vi "Crop Video Time.vi"() -> ()   [LabVIEW 2017]
uses:
  <vilib>/vision/NI_Vision_Development_Module.lvlib
  <vilib>/userdefined/High Color/IMAQdx.ctl
  <vilib>/vision/Image Controls.llb/IMAQ Image.ctl
  <vilib>/vision/Avi.llb/IMAQ AVI2 Refnum.ctl
  WEISS-Ultrasound-Frame-Grabber/LabVIEW/Controls/Position.ctl
  WEISS-Ultrasound-Frame-Grabber/LabVIEW/Controls/Orientation.ctl
  WEISS-Ultrasound-Frame-Grabber/LabVIEW/Controls/Rigid Body Info.ctl
  WEISS-Ultrasound-Frame-Grabber/LabVIEW/Controls/Refnums.ctl
  WEISS-Ultrasound-Frame-Grabber/LabVIEW/Controls/Room Dimensions.ctl
  WEISS-Ultrasound-Frame-Grabber/LabVIEW/Controls/Dimensions.ctl
  WEISS-Ultrasound-Frame-Grabber/LabVIEW/Controls/Frame Grabber Data.ctl
  WEISS-Ultrasound-Frame-Grabber/LabVIEW/Controls/Recording Settings.ctl
  WEISS-Ultrasound-Frame-Grabber/LabVIEW/Controls/Operator.ctl
  WEISS-Ultrasound-Frame-Grabber/LabVIEW/Controls/Operator Settings.ctl
panel:
  in  "Crop Outside":bool
  in  "Play":bool
  in  "Frame Slider":cluster{u32, u32, u32}(slide)={162, 79, 57} scale=0.0..179.0
  in  "Codec":u16(ring)=3 items=["Cinepak Codec by Radius", "Intel IYUV codec", "Microsoft Video 1", "FF Video Codec 1 (FFV1) (NI Vision)", "Motion JPEG (NI Vision)", "Y800 Uncompressed Grey Scale (NI Vision)", "YUV 4:2:0 Planar (NI Vision)"]
  out "Saving":bool
  in  "Display?":bool
  in  "Crop Inside":bool
  in  "Stop":bool
  out "Video path":path
  out "Crop ROI":i32[](array[numeric])
  in  "Frame Grabber Data":T1={"Camera Session"="", "Frame"=refnum, "AVI Refnum"=refnum, "Codecs"=[], "Frame number"=0, "Tracking File Refnum"=refnum, "Tick Count"=0, "Probe Object"=refnum, "Playback Probe Data"=[], "Rigid Body"={"Position"={"x (mm)"=0.0, "y (mm)"=0.0, "z (mm)"=0.0}, "Orientation"={"Pitch (rad)"=0.0, "Yaw (rad)"=0.0, "Roll (rad)"=0.0}, "Quaternion"={"qx"=0.0, "qy"=0.0, "qz"=0.0, "qw"=0.0}, "Tracked?"=FALSE}, "Total no frames playback"=0, "Video FPS"=0.0, "Camera connected?"=FALSE, "Scene"=refnum, "Cropped Frame"=refnum, "Tracker FPS"=0.0, "Crop ROI"=[], "Presentation Values"=[], "Elapsed time (ms)"=0, "Camera frames playback"=0, "Refnums"={"Live Refnum"=refnum, "Record Refnum"=refnum, "Recording Settings Refnum"=refnum, "Playback Refnum"=refnum, "Frame Slider Refnum"=refnum, "Pause Refnum"=refnum, "Home Refnum"=refnum, "Crop Refnum"=refnum, "Clear Crop Refnum"=refnum, "stop refnum"=refnum, "Playback Rate Refnum"=refnum, "Operator Settings Refnums"=refnum, "Presentation Refnum"=refnum, "Gestation Refnum"=refnum, "Connection Settings Refnum"=refnum}, "Dimensions"={"Probe Dimensions"={"Probe Width"=0.0, "Probe Depth"=1.0, "Probe Height"=0.0}, "Room Dimensions"={"Room Width"=0.0, "Room Depth"=0.0, "Room Height"=0.0}}}
  in  "Save":bool
  in  "Open":bool
  out "Frame":T3(plugin-control)
  # "Frame"
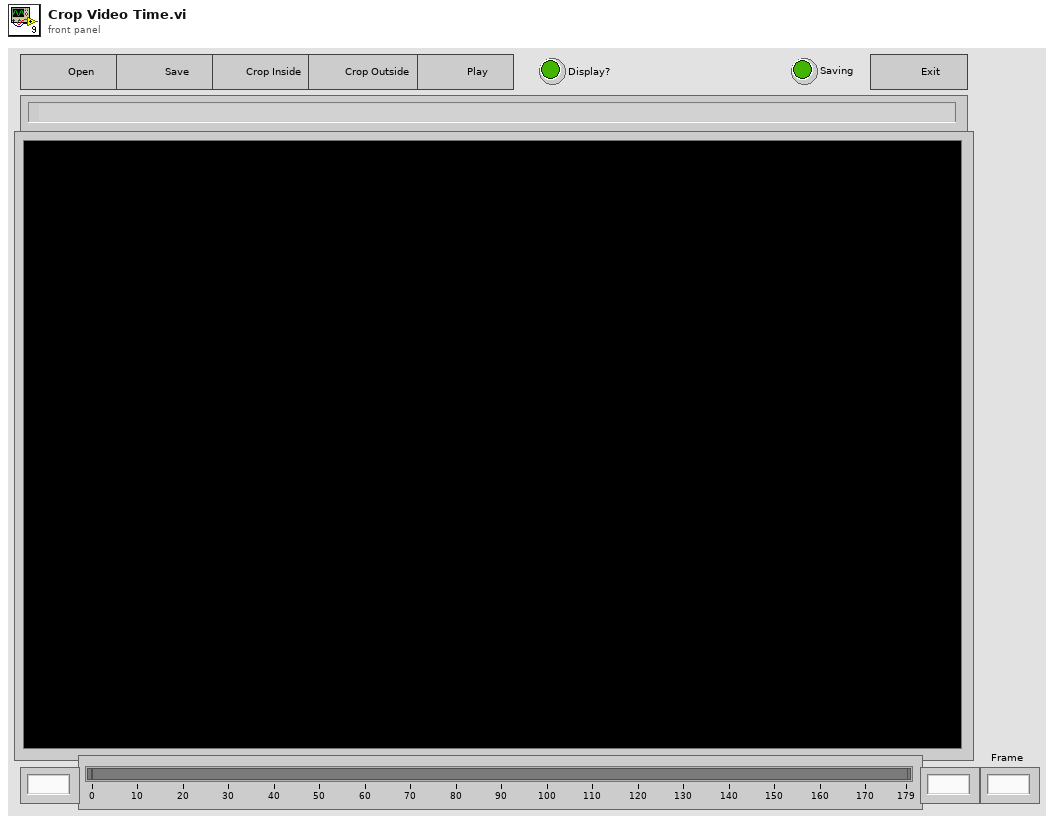
[diagram p1: front panel]
types:
  T1 = typedef "Frame Grabber Data.ctl" = cluster{"Camera Session":T2, "Frame":T3, "AVI Refnum":T4, "Codecs":string[], "Frame number":u32, "Tracking File Refnum":refnum<file>, "Tick Count":u32, "Probe Object":refnum<vi>, "Playback Probe Data":dbl[][], "Rigid Body":T5, "Total no frames playback":i32, "Video FPS":dbl, "Camera connected?":bool, "Scene":refnum<vi>, "Cropped Frame":T3, "Tracker FPS":dbl, "Crop ROI":i32[], "Presentation Values":string[], "Elapsed time (ms)":u32, "Camera frames playback":u32, "Refnums":T8, "Dimensions":T9}
  T2 = typedef "IMAQdx.ctl" = refnum<k21>
  T3 = typedef "IMAQ Image.ctl" = refnum<image>
  T4 = typedef "IMAQ AVI2 Refnum.ctl" = refnum<k20>
  T5 = typedef "Rigid Body Info.ctl" = cluster{"Position":T6, "Orientation":T7, "Quaternion":cluster{"qx":sgl, "qy":sgl, "qz":sgl, "qw":sgl}, "Tracked?":bool}
  T6 = typedef "Position.ctl" = cluster{"x (mm)":sgl, "y (mm)":sgl, "z (mm)":sgl}
  T7 = typedef "Orientation.ctl" = cluster{"Pitch (rad)":sgl, "Yaw (rad)":sgl, "Roll (rad)":sgl}
  T8 = typedef "Refnums.ctl" = cluster{"Live Refnum":refnum<vi>, "Record Refnum":refnum<vi>, "Recording Settings Refnum":refnum<vi>, "Playback Refnum":refnum<vi>, "Frame Slider Refnum":refnum<vi>, "Pause Refnum":refnum<vi>, "Home Refnum":refnum<vi>, "Crop Refnum":refnum<vi>, "Clear Crop Refnum":refnum<vi>, "stop refnum":refnum<vi>, "Playback Rate Refnum":refnum<vi>, "Operator Settings Refnums":refnum<vi>, "Presentation Refnum":refnum<vi>, "Gestation Refnum":refnum<vi>, "Connection Settings Refnum":refnum<vi>}
  T9 = typedef "Dimensions.ctl" = cluster{"Probe Dimensions":cluster{"Probe Width":sgl, "Probe Depth":sgl, "Probe Height":sgl}, "Room Dimensions":T10}
  T10 = typedef "Room Dimensions.ctl" = cluster{"Room Width":dbl, "Room Depth":dbl, "Room Height":dbl}
  T11 = enum16{"Init", "Wait", "Load", "Playback", "Crop Inside", "Crop Outside", "Shutdown"}
  T12 = enum8{"Enabled", "Disabled", "Disabled and Grayed Out"}
  T13 = typedef "Image Type" = u32
  T14 = enum16{"open", "replace", "create", "open or create", "replace or create", "replace or create with confirmation"}
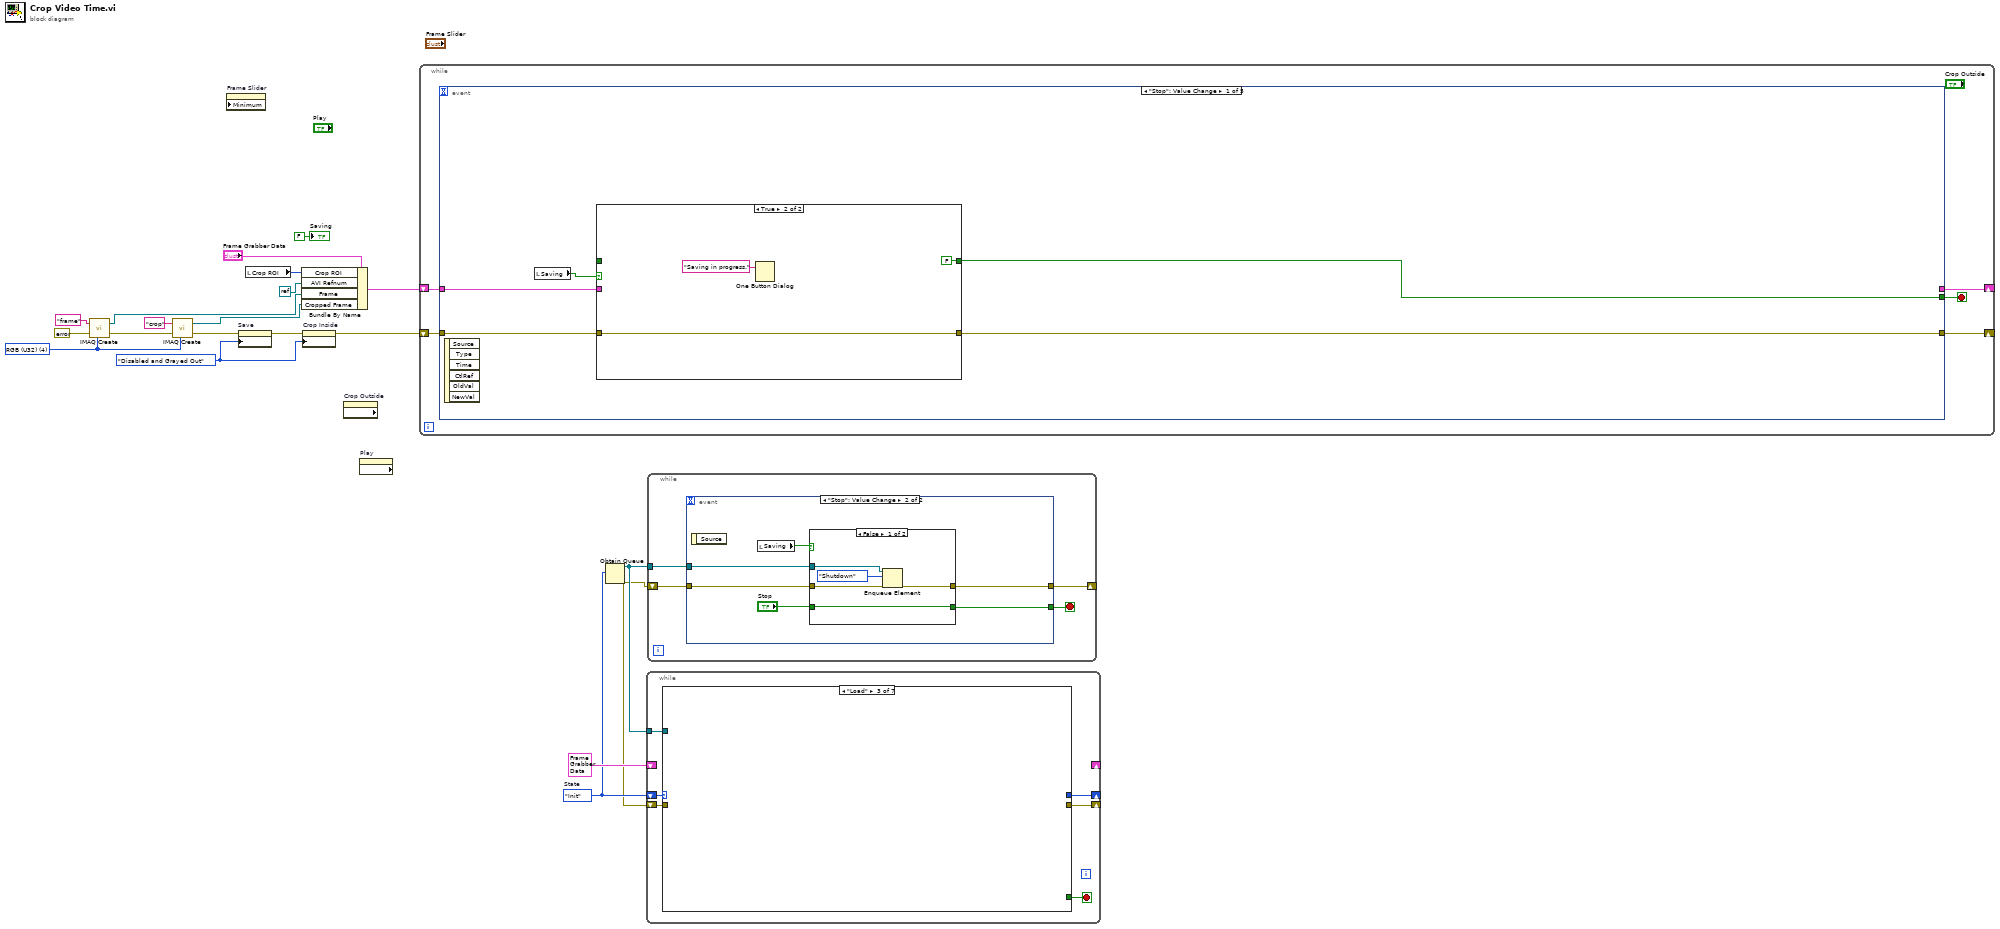
[diagram p0: block diagram]
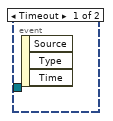
[diagram p2: hidden frame]
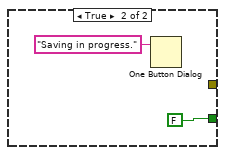
[diagram p3: hidden frame]
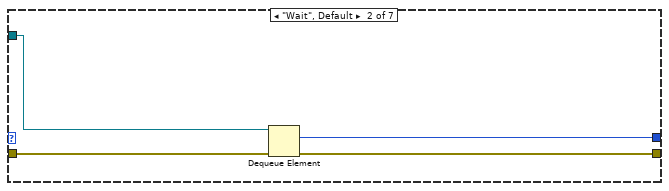
[diagram p5: hidden frame]
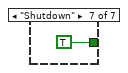
[diagram p9: hidden frame]
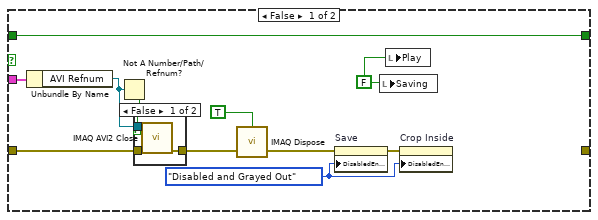
[diagram p10: hidden frame]
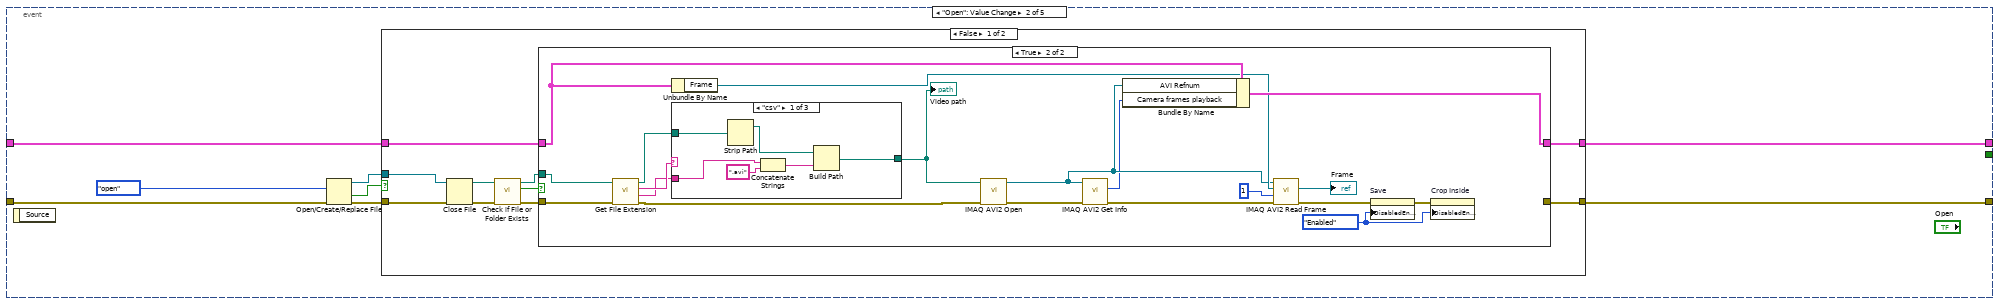
[diagram p12: hidden frame]
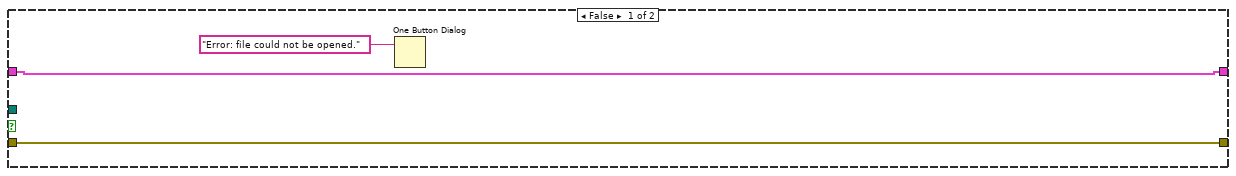
[diagram p13: hidden frame]
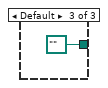
[diagram p15: hidden frame]
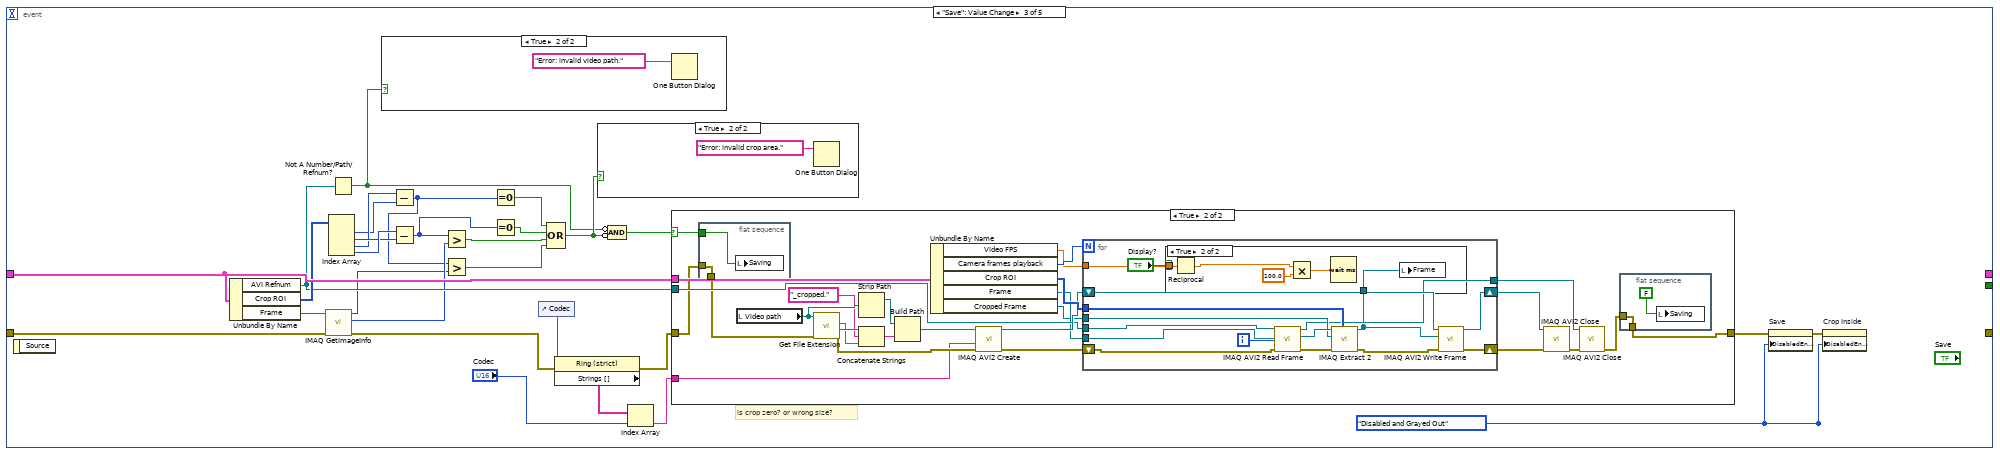
[diagram p17: hidden frame]
diagram:
  w3 = T11."Init"  # State
  w7 = T12."Disabled and Grayed Out" ("Disabled")
  w12 = T13 4 items=["Grayscale (U8)", "Grayscale (I16)", "Grayscale (SGL)", "Complex (CSG)", "RGB (U32)", "HSL (U32)", "RGB (U64)", "Grayscale (U16)"] ("Image Type")
  n1 = call "IMAQ Create"("Image Name"="frame", "Image Type"=w12, "error in (no error)"=errorcluster {"status"=FALSE, "code"=0, "source"=""}) -> ("New Image"=w15:T3, "error out"=w13:errorcluster)  [unwired: 2 in]
  n2 = call "IMAQ Create"("Image Name"="crop", "Image Type"=w12, "error in (no error)"=w13) -> ("New Image"=w16:T3, "error out"=w9:errorcluster)  [unwired: 2 in]
  n3 = property on="Frame Slider" class="Slide (strict)" props=["Minimum"]() -> ()  [unwired: 3 in, 2 out]
  n4 = property on="Save" class="Bool"(error in=w9, "DisabledEnum"=w7) -> (error out=w8:errorcluster)  [unwired: 1 in, 1 out]
  n5 = local read "Crop ROI"() -> (w10:i32[])
  n6 = Bundle By Name(cluster="Frame Grabber Data", "Crop ROI"=w10, "AVI Refnum"=refnum<k0> refnum, "Frame"=w15, "Cropped Frame"=w16) -> (w19:T1)
  n7 = property on="Crop Inside" class="Bool"(error in=w8, "DisabledEnum"=w7) -> (error out=w5:errorcluster)  [unwired: 1 in, 1 out]
  n8 = property on="Crop Outside" class="Bool" props=["DisabledEnum"]() -> ()  [unwired: 2 in, 3 out]
  n9 = property on="Play" class="Bool (strict)" props=["DisabledEnum"]() -> ()  [unwired: 2 in, 3 out]
  n10 = while {
    shift-right: [w22] -> _
    shift-left: w19 -> [w23]
    shift-right: [w21] -> _
    shift-left: w5 -> [w24]
    stop <- w25 stop-if-true
    n11 = event shown="[0] \"Stop\": Value Change" {
      selector: _ -> [_ _ _ _ _]
      dyn-events: _ -> [_ _ _ _ _]
      timeout: _ -> [_ _ _ _ _]
      tunnel: [w26 _ _ _ _] -> w25
      tunnel: w24 -> [w30 w57 w116 w189 w193]
      tunnel: w23 -> [w29 w52 w129 w190 w196]
      tunnel: [_ w51 _ w188 w191] -> w22
      tunnel: [w28 w50 w108 w185 w192] -> w21
      event "Stop": Value Change {
        n12 = event-data() -> ()  [unwired: 1 in, 6 out]
        n13 = local read "Saving"() -> (w27:bool)
        n14 = case shown="True" w27 {
          tunnel: w30 -> [w42 w48]
          tunnel: w29 -> [w41 _]
          tunnel: [w37 w48] -> w28
          tunnel: _ -> [w32 _]
          tunnel: [w32 FALSE ("Stop")] -> w26
          frame False {
            w31 = FALSE
            w35 = T12."Disabled and Grayed Out" ("Disabled")
            n15 = Unbundle By Name(w41) -> ("AVI Refnum"=w34:T4)
            n16 = Not A Number/Path/Refnum?(number/path/refnum=w34) -> (NaN/Path/Refnum?=w33:bool)
            n17 = case shown="False" w33 {
              tunnel: w42 -> [w45 w46]
              tunnel: [w44 w46] -> w39
              tunnel: w34 -> [w43 _]
              frame False {
                n18 = call "IMAQ AVI2 Close"("error in (no error)"=w45, "AVI Refnum"=w43) -> ("error out"=w44:errorcluster)  [unwired: 9 in]
              }
              frame True {
              }
            }
            n19 = call "IMAQ Dispose"("All Images? (No)"=TRUE, "error in (no error)"=w39) -> ("error out"=w38:errorcluster)  [unwired: 4 in]
            n20 = property on="Save" class="Bool"(error in=w38, "DisabledEnum"=w35) -> (error out=w36:errorcluster)  [unwired: 1 in, 1 out]
            n21 = local write "Saving"(w31) -> ()
            n22 = local write "Play"(w31) -> ()
            n23 = property on="Crop Inside" class="Bool"(error in=w36, "DisabledEnum"=w35) -> ()  [unwired: 1 in, 2 out]
          }
          frame True {
            n24 = One Button Dialog(message="Saving in progress.") -> ()  [unwired: 1 in, 1 out]
          }
        }
      }
      event "Open": Value Change {
        n25 = event-data() -> ()  [unwired: 1 in, 1 out]
        n26 = Open/Create/Replace File(error in=w57, operation (0:open)=T14."open") -> (refnum out=w53:refnum<file>, cancelled=w56:bool, error out=w54:errorcluster)  [unwired: 4 in]
        n27 = case shown="False" w56 {
          tunnel: w54 -> [w64 w98]
          tunnel: w53 -> [w65 _]
          tunnel: w52 -> [w61 w99]
          tunnel: [w60 w99] -> w51
          tunnel: [w58 w98] -> w50
          frame False {
            n28 = Close File(refnum=w65, error in=w64) -> (path=w62:path, error out=w63:errorcluster)
            n29 = call <vilib>:"Check if File or Folder Exists.vi"("error in (no error)"=w63, "path"=w62) -> ("error out"=w67:errorcluster, "file or folder exists?"=w59:bool, "dup path"=w66:path)  [unwired: 7 in]
            n30 = case shown="True" w59 {
              tunnel: w67 -> [w69 w77]
              tunnel: w66 -> [_ w73]
              tunnel: w61 -> [w70 w88]
              tunnel: [w70 w89] -> w60
              tunnel: [w69 _] -> w58
              frame False {
                n31 = One Button Dialog(message="Error: file could not be opened.") -> ()  [unwired: 1 in, 1 out]
              }
              frame True {
                w78 = T12."Enabled" ("Disabled")
                n32 = call <vilib>:"Get File Extension.vi"("error in (no error)"=w77, "file"=w73) -> ("error out"=w76:errorcluster, "filename without extension"=w74:string, "lowercase file extension"=w75:string, "dup file"=w72:path)  [unwired: 5 in, 1 out]
                n33 = Unbundle By Name(w88) -> ("Frame"=w87:T3)
                n34 = case shown="\"csv\"" w75 {
                  tunnel: w74 -> [w95 _ _]
                  tunnel: [w90 w96 path "" ("dup file")] -> w71
                  tunnel: w72 -> [w91 w96 _]
                  frame "csv" {
                    n35 = Strip Path(path=w91) -> (stripped path=w93:path)  [unwired: 1 out]
                    n36 = Concatenate Strings(w95, ".avi" ("string")) -> (w92:string)
                    n37 = Build Path(base path=w93, name or relative path=w92) -> (appended path=w90:path)
                  }
                  frame "avi" {
                  }
                  frame Default {
                  }
                }
                "Video path" <- w71
                n38 = call "IMAQ AVI2 Open"("error in (no error)"=w76, "AVI File Path"=w71) -> ("error out"=w83:errorcluster, "AVI Refnum"=w84:T4)  [unwired: 8 in]
                n39 = call "IMAQ AVI2 Get Info"("error in (no error)"=w83, "AVI Refnum"=w84) -> ("error out"=w82:errorcluster, "Number of Frames"=w81:u32)  [unwired: 5 in, 3 out]
                n40 = Bundle By Name(cluster=w88, "AVI Refnum"=w84, "Camera frames playback"=w81) -> (w89:T1)
                n41 = call "IMAQ AVI2 Read Frame"("error in (no error)"=w82, "Frame Number"=u32 1, "Image"=w87, "AVI Refnum"=w84) -> ("error out"=w80:errorcluster, "Image Out"=→"Frame":T3)  [unwired: 5 in, 1 out]
                n42 = property on="Save" class="Bool"(error in=w80, "DisabledEnum"=w78) -> (error out=w79:errorcluster)  [unwired: 1 in, 1 out]
                n43 = property on="Crop Inside" class="Bool"(error in=w79, "DisabledEnum"=w78) -> ()  [unwired: 1 in, 2 out]
              }
            }
          }
          frame True {
          }
        }
      }
      event "Save": Value Change {
        w106 = T12."Disabled and Grayed Out" ("Disabled")
        # "is crop zero? or wrong size?"
        n44 = event-data() -> ()  [unwired: 1 in, 1 out]
        n45 = Unbundle By Name(w129) -> ("AVI Refnum"=w117:T4, "Crop ROI"=w122:i32[], "Frame"=w115:T3)
        n46 = call "IMAQ GetImageInfo"("error in (no error)"=w116, "Image"=w115) -> ("error out"=w105:errorcluster, "Y Resolution"=w114:i32, "X Resolution"=w112:i32)  [unwired: 2 in, 5 out]
        n47 = Index Array(array=w122) -> (element #1=w123:i32, element #2=w125:i32, element #3=w124:i32, element #4=w126:i32)  [unwired: 4 in]
        n48 = Not A Number/Path/Refnum?(number/path/refnum=w117) -> (NaN/Path/Refnum?=w118:bool)
        n49 = case shown="True" w118 {
          frame False {
          }
          frame True {
            n50 = One Button Dialog(message="Error: invalid video path.") -> ()  [unwired: 1 in, 1 out]
          }
        }
        n51 = Subtract(x=w124, y=w123) -> (x-y=w111:i32)
        n52 = Subtract(x=w126, y=w125) -> (x-y=w109:i32)
        n53 = Greater?(x=w109, y=w114) -> (0:w113:bool)
        n54 = Greater?(x=w111, y=w112) -> (0:w110:bool)
        n55 = Equal To 0?(x=w111) -> (x = 0?=w127:bool)
        n56 = Equal To 0?(x=w109) -> (x = 0?=w128:bool)
        n57 = control-ref of="Codec"() -> (w103:refnum<vi>)
        n58 = Compound Arithmetic op=OR(w127, w128, w113, w110) -> (w119:bool)
        n59 = property class="Ring (strict)"(reference=w103, error in=w105) -> (error out=w104:errorcluster, "Strings []"=w101:string[])  [unwired: 1 out]
        n60 = case shown="True" w119 {
          frame False {
          }
          frame True {
            n61 = One Button Dialog(message="Error: invalid crop area.") -> ()  [unwired: 1 in, 1 out]
          }
        }
        n62 = Compound Arithmetic op=AND(invert w118, invert w119) -> (w120:bool)
        n63 = Index Array(array=w101, index="Codec") -> (element=w100:string)
        n64 = case shown="True" w120 {
          selector: w120 -> [_ w138]
          tunnel: w129 -> [_ w159]
          tunnel: w117 -> [_ w146]
          tunnel: [w132 w134] -> w121
          tunnel: w104 -> [w132 w137]
          tunnel: w100 -> [_ w133]
          frame False {
          }
          frame True {
            n65 = flat-sequence {
              tunnel: w138 -> [w163]
              tunnel: w137 -> [w162]
              tunnel: [w162] -> w136
              frame #0 {
                n66 = local write "Saving"(w163) -> ()
              }
            }
            n67 = local read "Video path"() -> (w154:path)
            n68 = call <vilib>:"Get File Extension.vi"("error in (no error)"=w136, "file"=w154) -> ("error out"=w155:errorcluster, "filename without extension"=w152:string, "lowercase file extension"=w150:string)  [unwired: 5 in, 2 out]
            n69 = Strip Path(path=w154) -> (stripped path=w153:path)  [unwired: 1 out]
            n70 = Concatenate Strings(w152, "_cropped." ("string"), w150) -> (w149:string)
            n71 = Build Path(base path=w153, name or relative path=w149) -> (appended path=w148:path)
            n72 = Unbundle By Name(w159) -> ("Video FPS"=w139:dbl, "Camera frames playback"=w158:u32, "Crop ROI"=w157:i32[], "Frame"=w145:T3, "Cropped Frame"=w144:T3)
            n73 = call "IMAQ AVI2 Create"("error in (no error)"=w155, "Codec"=w133, "AVI Path"=w148) -> ("error out"=w147:errorcluster, "AVI Refnum"=w156:T4)  [unwired: 7 in]
            n74 = for {
              N: w158 -> [_]
              shift-right: [w174] -> w143
              shift-left: w147 -> [w178]
              tunnel: w157 -> [w177]
              tunnel: w146 -> [w173]
              tunnel: w145 -> [w172]
              tunnel: w144 -> [w170]
              shift-right: [w169] -> w142
              shift-left: w156 -> [w176]
              tunnel: [w168] -> w140
              tunnel: w139 -> [w165]
              i -> [w179]
              n75 = call "IMAQ AVI2 Read Frame"("error in (no error)"=w178, "Frame Number"=w179, "Image"=w172, "AVI Refnum"=w173) -> ("error out"=w166:errorcluster, "Image Out"=w171:T3, "AVI Refnum (duplicate)"=w168:T4)  [unwired: 5 in]
              n76 = call "IMAQ Extract 2"("Optional Rectangle"=w177, "error in (no error)"=w166, "Image Dst"=w170, "Image Src"=w171) -> ("error out"=w175:errorcluster, "Image Dst Out"=w167:T3)  [unwired: 6 in]
              n77 = case shown="True" "Display?" {
                tunnel: w167 -> [_ w184]
                tunnel: w165 -> [_ w183]
                frame False {
                }
                frame True {
                  n78 = Reciprocal(x=w183) -> (1/x=w182:dbl)
                  n79 = Multiply(x=w182, y=100.0) -> (x*y=w180:dbl)
                  n80 = Wait (ms)(milliseconds to wait=w180) -> ()  [unwired: 1 out]
                  n81 = local write "Frame"(w184) -> ()
                }
              }
              n82 = call "IMAQ AVI2 Write Frame"("error in (no error)"=w175, "Image"=w167, "AVI Refnum"=w176) -> ("error out"=w174:errorcluster, "AVI Refnum (duplicate)"=w169:T4)  [unwired: 6 in, 1 out]
            }
            n83 = call "IMAQ AVI2 Close"("error in (no error)"=w143, "AVI Refnum"=w142) -> ("error out"=w141:errorcluster)  [unwired: 9 in]
            n84 = call "IMAQ AVI2 Close"("error in (no error)"=w141, "AVI Refnum"=w140) -> ("error out"=w135:errorcluster)  [unwired: 9 in]
            n85 = flat-sequence {
              tunnel: w135 -> [w161]
              tunnel: [w161] -> w134
              frame #0 {
                n86 = local write "Saving"(FALSE) -> ()
              }
            }
          }
        }
        n87 = property on="Save" class="Bool"(error in=w121, "DisabledEnum"=w106) -> (error out=w107:errorcluster)  [unwired: 1 in, 1 out]
        n88 = property on="Crop Inside" class="Bool"(error in=w107, "DisabledEnum"=w106) -> ()  [unwired: 1 in, 2 out]
      }
      event "Crop Inside": Value Change {
        n89 = event-data() -> ()  [unwired: 1 in, 1 out]
        n90 = call "Set Crop ROI.vi"("error in (no error)"=w189, "Frame Grabber Data in"=w190) -> ("error out"=w185:errorcluster, "Crop ROI"=→"Crop ROI":i32[], "Image Out"=w187:T3, "Frame Grabber Data out"=w188:T1)  [unwired: 6 in]
        n91 = local write "Frame"(w187) -> ()
      }
      event #4 (no event record) {
        n92 = event-data() -> ()  [unwired: 1 in, 1 out]
        n93 = call "Clear Crop ROI.vi"("error in (no error)"=w193, "Frame Grabber Data in"=w196) -> ("error out"=w192:errorcluster, "Image Out"=w195:T3, "Crop ROI"=w194:i32[], "Frame Grabber Data out"=w191:T1)  [unwired: 6 in]
        n94 = local write "Frame"(w195) -> ()
        n95 = local write "Crop ROI"(w194) -> ()
      }
    }
  }
  n96 = Obtain Queue(element data type=w3) -> (queue out=w2:refnum<queue>, error out=w1:errorcluster)  [unwired: 4 in, 1 out]
  n97 = while {
    shift-right: _ -> [_]
    shift-left: T1 {"Camera Session"="", "Frame"=refnum, "AVI Refnum"=refnum, "Codecs"=[], "Frame number"=0, "Tracking File Refnum"=refnum, "Tick Count"=0, "Probe Object"=refnum, "Playback Probe Data"=[], "Rigid Body"={"Position"={"x (mm)"=0.0, "y (mm)"=0.0, "z (mm)"=0.0}, "Orientation"={"Pitch (rad)"=0.0, "Yaw (rad)"=0.0, "Roll (rad)"=0.0}, "Quaternion"={"qx"=0.0, "qy"=0.0, "qz"=0.0, "qw"=0.0}, "Tracked?"=FALSE}, "Total no frames playback"=0, "Video FPS"=0.0, "Camera connected?"=FALSE, "Scene"=refnum, "Cropped Frame"=refnum, "Tracker FPS"=0.0, "Crop ROI"=[], "Presentation Values"=[], "Elapsed time (ms)"=0, "Camera frames playback"=0, "Refnums"={"Live Refnum"=refnum, "Record Refnum"=refnum, "Recording Settings Refnum"=refnum, "Playback Refnum"=refnum, "Frame Slider Refnum"=refnum, "Pause Refnum"=refnum, "Home Refnum"=refnum, "Crop Refnum"=refnum, "Clear Crop Refnum"=refnum, "stop refnum"=refnum, "Playback Rate Refnum"=refnum, "Operator Settings Refnums"=refnum, "Presentation Refnum"=refnum, "Gestation Refnum"=refnum, "Connection Settings Refnum"=refnum}, "Dimensions"={"Probe Dimensions"={"Probe Width"=0.0, "Probe Depth"=1.0, "Probe Height"=0.0}, "Room Dimensions"={"Room Width"=0.0, "Room Depth"=0.0, "Room Height"=0.0}}} ("Frame Grabber Data 2") -> [_]
    tunnel: w2 -> [w200]
    shift-right: [w198] -> _
    shift-left: w1 -> [w199]
    shift-right: [w197] -> _
    shift-left: w3 -> [w202]
    stop <- w201 stop-if-true
    n98 = case shown="\"Load\"" w202 {
      tunnel: [_ _ _ _ _ _ TRUE] -> w201
      tunnel: w200 -> [_ w206 _ _ _ _ _]
      tunnel: w199 -> [_ w205 _ _ _ _ _]
      tunnel: [_ w204 _ _ _ _ _] -> w198
      tunnel: [_ w203 _ _ _ _ _] -> w197
      frame "Init" {
      }
      frame "Wait", Default {
        n99 = Dequeue Element(queue=w206, error in (no error)=w205) -> (element=w203:T11, error out=w204:errorcluster)  [unwired: 1 in, 2 out]
      }
      frame "Load" {
      }
      frame "Playback" {
      }
      frame "Crop Inside" {
      }
      frame "Crop Outside" {
      }
      frame "Shutdown" {
      }
    }
  }
  n100 = while {
    tunnel: w2 -> [w210]
    shift-right: [w208] -> _
    shift-left: w1 -> [w209]
    stop <- w211 stop-if-true
    n101 = event shown="[1] \"Stop\": Value Change" {
      selector: _ -> [_ _]
      dyn-events: _ -> [_ _]
      timeout: _ -> [_ _]
      tunnel: [_ w215] -> w211
      tunnel: w210 -> [_ w214]
      tunnel: w209 -> [_ w213]
      tunnel: [_ w212] -> w208
      event Timeout {
        n102 = event-data() -> ()  [unwired: 1 in, 3 out]
      }
      event "Stop": Value Change {
        n103 = event-data() -> ()  [unwired: 1 in, 1 out]
        n104 = local read "Saving"() -> (w217:bool)
        n105 = case shown="False" w217 {
          tunnel: "Stop" -> [w222 _]
          tunnel: [w222 FALSE] -> w215
          tunnel: w214 -> [w221 _]
          tunnel: w213 -> [w219 _]
          tunnel: [w218 _] -> w212
          frame False {
            n106 = Enqueue Element(queue=w221, element=T11."Shutdown", error in (no error)=w219) -> (error out=w218:errorcluster)  [unwired: 1 in, 2 out]
          }
          frame True {
            n107 = One Button Dialog(message="Saving in progress.") -> ()  [unwired: 1 in, 1 out]
          }
        }
      }
    }
  }
  "Saving" <- FALSE ("Saving")
